vi "Set Control Data.vi"(8 "error in (no error)":errorcluster, 10 "Control Data":T1[](array[typedef]), 11 "Test Case in":refnum<class "Test Case.lvclass">) -> (0 "error out":errorcluster, 3 "Test Case out":refnum<class "Test Case.lvclass">)   [LabVIEW 2017, in "Test Case.lvclass"]
uses:
  Test Case.lvclass
  ControlData.ctl
  Test Case.lvclass/Test Case.ctl
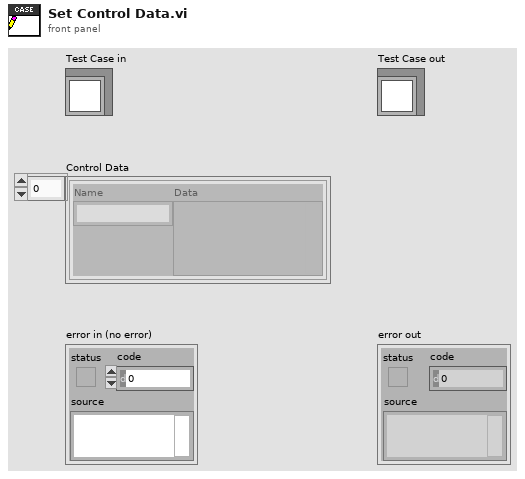
[diagram p1: front panel]
types:
  T1 = typedef "ControlData.ctl" = cluster{"Name":string, "Data":variant}
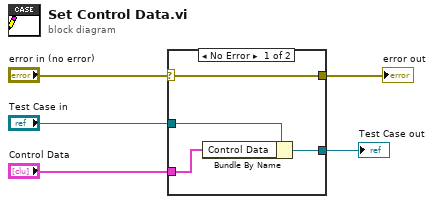
[diagram p0: block diagram]
diagram:
  n1 = case shown="No Error" "error in (no error)" {
    selector: "error in (no error)" -> [w9 w10]
    tunnel: [w9 w10] -> w4
    tunnel: [w7 w11] -> w2
    tunnel: "Test Case in" -> [w8 w11]
    tunnel: "Control Data" -> [w6 _]
    frame No Error {
      n2 = Bundle By Name(cluster=w8, "Control Data"=w6) -> (w7:refnum<class "Test Case.lvclass">)
    }
    frame Error {
    }
  }
  "error out" <- w4
  "Test Case out" <- w2
